vi "SetParam.vi"(8 "error in (no error)":errorcluster caption="entrée d'erreur (pas d'erreur)", 10 "silhouette_samples":cluster{"metric":string}={"metric"="euclidean"}, 11 "Silhouette_Samples.lvclass":refnum<class "Silhouette_Samples.lvclass">) -> (0 "error out":errorcluster caption="sortie d'erreur", 3 "Silhouette_Samples.lvclass":refnum<class "Silhouette_Samples.lvclass">)   [LabVIEW 2020, in "Silhouette_Samples.lvclass"]
doc: "Set Parameters"
uses:
  Silhouette_Samples.lvclass
  Silhouette_Samples.lvclass/Silhouette_Samples.ctl
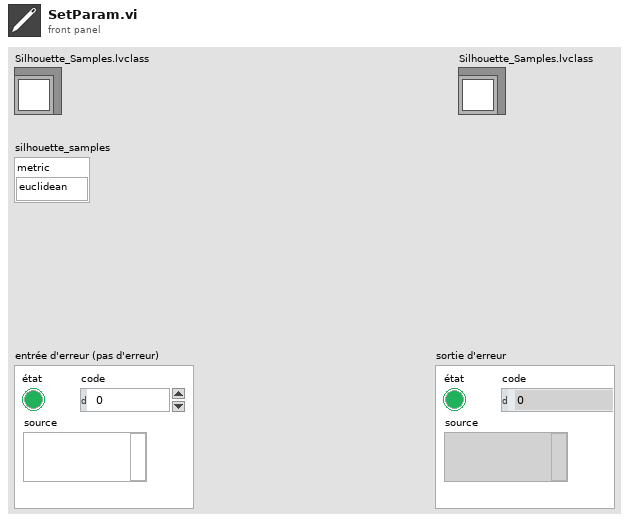
[diagram p1: front panel]
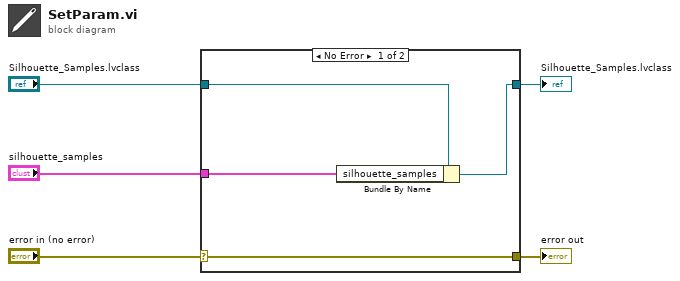
[diagram p0: block diagram]
diagram:
  n1 = case shown="No Error" "error in (no error)" {
    selector: "error in (no error)" -> [w9 w10]
    tunnel: [w9 w10] -> w4
    tunnel: [w7 w11] -> w2
    tunnel: "Silhouette_Samples.lvclass" -> [w8 w11]
    tunnel: "silhouette_samples" -> [w6 _]
    frame No Error {
      n2 = Bundle By Name(cluster=w8, "silhouette_samples"=w6) -> (w7:refnum<class "Silhouette_Samples.lvclass">)
    }
    frame Error {
    }
  }
  "error out" <- w4
  "Silhouette_Samples.lvclass" <- w2
